vi "Check if Plugin Name in Library.vi"(0 "project exists?":bool, 5 "library name":string, 7 "library names":string[](array[string]), 11 "error in":errorcluster) -> (4 "found":bool, 15 "error out":errorcluster)   [LabVIEW 2021, in "Converter.lvlib"]
uses:
  Converter.lvlib
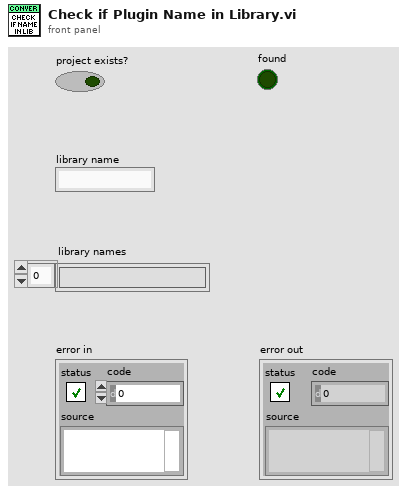
[diagram p1: front panel]
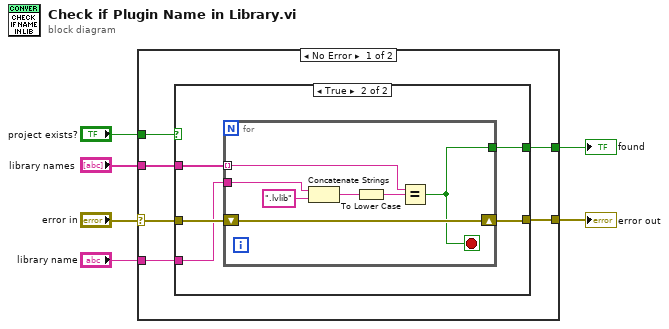
[diagram p0: block diagram]
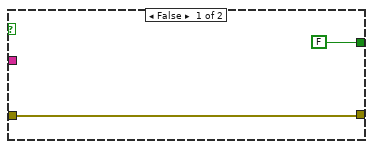
[diagram p2: hidden frame]
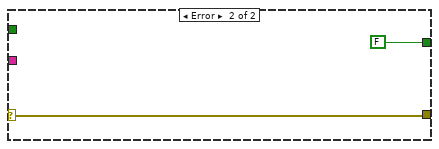
[diagram p3: hidden frame]
diagram:
  n1 = case shown="No Error" "error in" {
    selector: "error in" -> [w10 w27]
    tunnel: "library name" -> [w12 _]
    tunnel: [w11 w27] -> w4
    tunnel: [w9 FALSE] -> w3
    tunnel: "project exists?" -> [w8 _]
    tunnel: "library names" -> [w7 _]
    frame No Error {
      n2 = case shown="True" w8 {
        tunnel: w12 -> [_ w18]
        tunnel: [w13 w17] -> w11
        tunnel: w10 -> [w13 w19]
        tunnel: [FALSE w15] -> w9
        tunnel: w7 -> [_ w16]
        frame False {
        }
        frame True {
          n3 = for {
            tunnel: w18 -> [w26]
            shift-right: [w24] -> w17
            shift-left: w19 -> [w24]
            tunnel: w16 -> [w21] mode=indexing
            tunnel: [w20] -> w15
            stop <- w20 stop-if-true
            n4 = Concatenate Strings(w26, ".lvlib" ("string")) -> (w23:string)
            n5 = To Lower Case(string=w23) -> (all lower case string=w22:string)
            n6 = Equal?(x=w21, y=w22) -> (x = y?=w20:bool)
          }
        }
      }
    }
    frame Error {
    }
  }
  "error out" <- w4
  "found" <- w3
